vi "SubVI_HighPassFilter.vi"(7 "Interpolant Size":dbl, 8 "error in (no error)":errorcluster, 9 "high cutoff freq":dbl, 10 "EEG Desired Frequency":dbl, 11 "Channel in":T1) -> (0 "error out":errorcluster, 3 "Channel out":T1)   [LabVIEW 2020]
uses:
  <extravilib>/ChannelInstances/Stream-a[.](dbl)/)Channel.ctl
  <vilib>/Analysis/3filter.llb/Filter Passband Type.ctl
  <extravilib>/ChannelInstances/Stream-a[.](dbl)/EndpointRead.vi
  <extravilib>/ChannelInstances/Stream-a[.](dbl)/Endpoint.vi
  Global 1.vi
  <extravilib>/ChannelInstances/Stream-a[.](dbl)/)Channel.vi
  <resource>/ChannelSupport/_ChannelSupport/WaitIfNeeded.vi
  <vilib>/Analysis/NI_AALBase.lvlib
  <vilib>/ptbypt/NI_PtbyPt.lvlib
  <extravilib>/ChannelInstances/Stream-a[.](dbl).lvlib
panel:
  out "Waveform Chart 2":dbl(graph)
  out "Waveform Chart":dbl(graph)
  in  "index 2":i32
  in  "index":i32
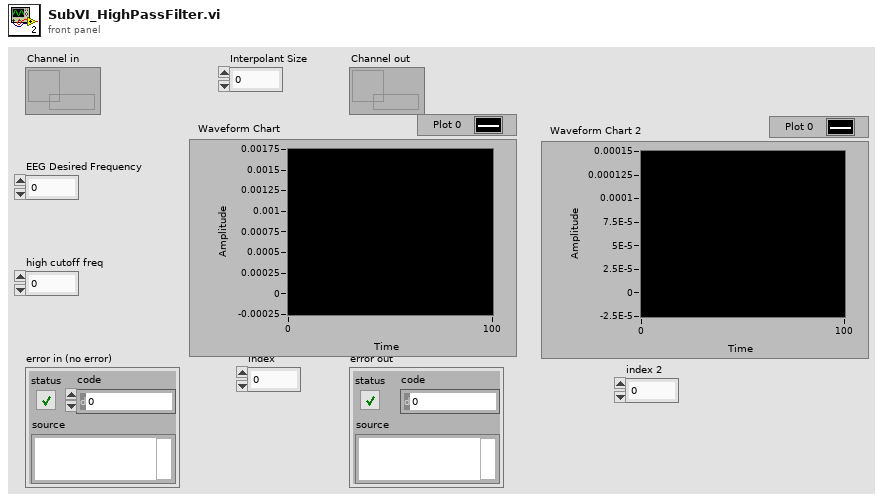
[diagram p1: front panel]
types:
  T1 = typedef "Stream-a[.](dbl).lvlib/)Channel.ctl" = refnum<queue>
  T2 = typedef "NI_AALBase.lvlib/Filter Passband Type.ctl" = enum32{"Lowpass", "Highpass", "Bandpass", "Bandstop"}
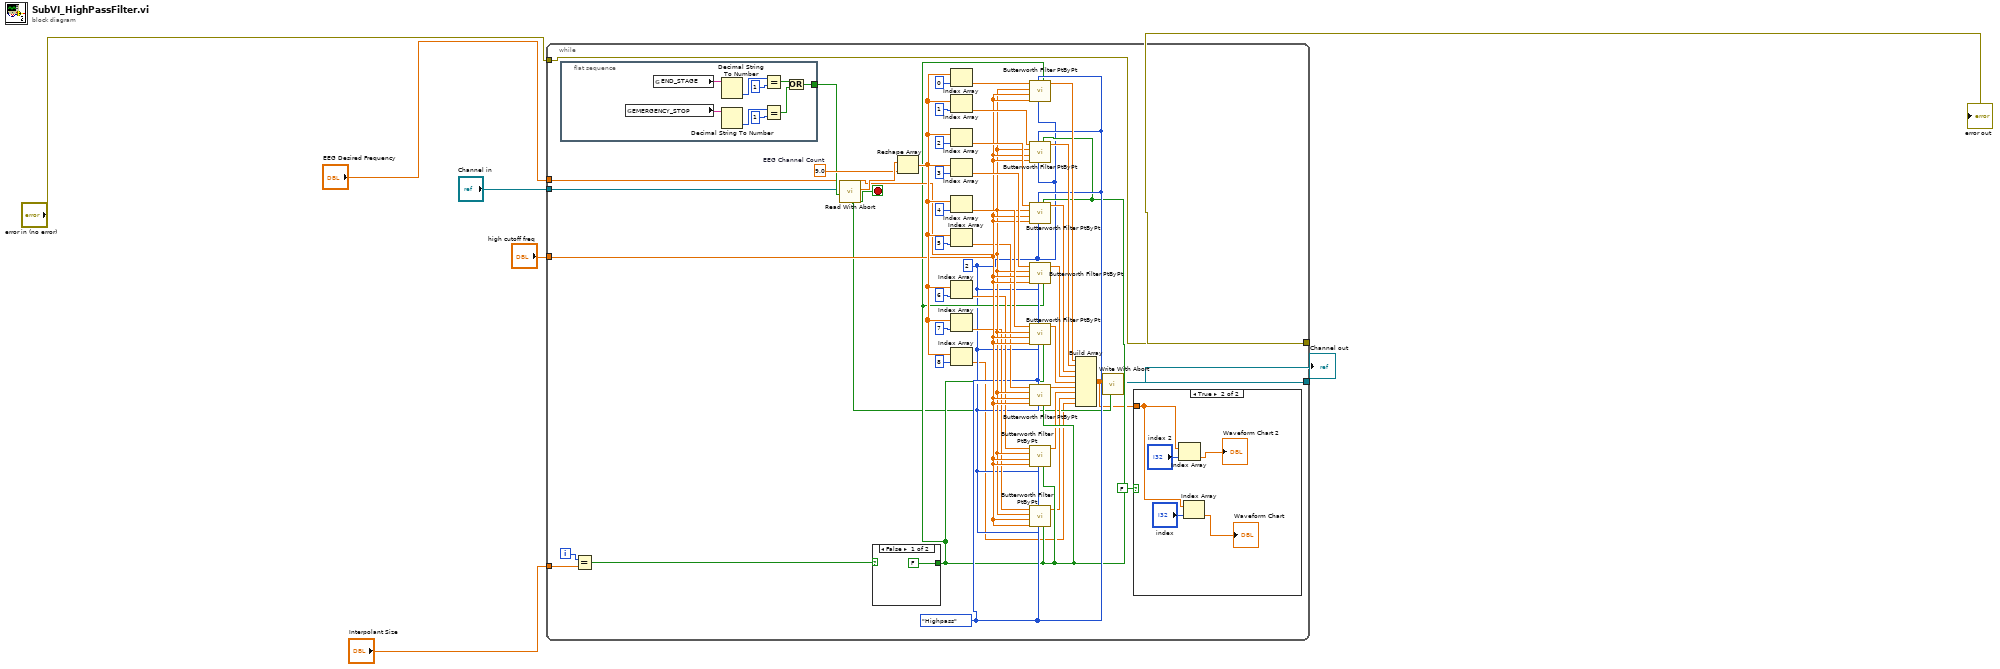
[diagram p0: block diagram]
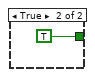
[diagram p3: hidden frame]
diagram:
  n1 = while {
    tunnel: "Channel in" -> [w29]
    tunnel: "Interpolant Size" -> [w37]
    tunnel: "EEG Desired Frequency" -> [w22]
    tunnel: "error in (no error)" -> [w30]
    tunnel: [w30] -> w7
    tunnel: "high cutoff freq" -> [w23]
    tunnel: [w11] -> w5
    i -> [w38]
    stop <- w12 stop-if-true
    w32 = 9.0  # EEG Channel Count
    w16 = 2 ("order")
    w18 = Filter_Passband_Type."Highpass" ("filter type")
    n2 = flat-sequence {
      tunnel: [w57] -> w31
      frame #0 {
        n3 = global read "Global 1.vi" "EMERGENCY_STOP"() -> (w60:string)
        n4 = global read "Global 1.vi" "END_STAGE"() -> (w65:string)
        n5 = Decimal String To Number(string=w65) -> (number=w64:i32)  [unwired: 2 in, 1 out]
        n6 = Decimal String To Number(string=w60) -> (number=w62:i32)  [unwired: 2 in, 1 out]
        n7 = Equal?(x=w64, y=1) -> (x = y?=w58:bool)
        n8 = Equal?(x=w62, y=1) -> (x = y?=w59:bool)
        n9 = Or(x=w58, y=w59) -> (x .or. y?=w57:bool)
      }
    }
    n10 = Equal?(x=w38, y=w37) -> (x = y?=w36:bool)
    n11 = call <extravilib>:"Read With Abort.vi"("abort"=w31, "channel"=w29) -> ("element"=w39:dbl[], "aborted?"=w12:bool)  [unwired: 4 in, 4 out]
    n12 = case shown="False" w36 {
      tunnel: [FALSE ("init/cont (init:F)") TRUE ("init/cont (init:F)")] -> w17
      frame False {
      }
      frame True {
      }
    }
    n13 = Reshape Array(w39, w32) -> (w24:dbl[])
    n14 = Index Array(array=w24, index=0 ("disabled index (col)")) -> (element=w48:dbl)
    n15 = Index Array(array=w24, index=1 ("disabled index (col)")) -> (element=w49:dbl)
    n16 = Index Array(array=w24, index=2 ("disabled index (col)")) -> (element=w50:dbl)
    n17 = Index Array(array=w24, index=3 ("disabled index (col)")) -> (element=w51:dbl)
    n18 = Index Array(array=w24, index=4 ("disabled index (col)")) -> (element=w35:dbl)
    n19 = Index Array(array=w24, index=5 ("disabled index (col)")) -> (element=w21:dbl)
    n20 = Index Array(array=w24, index=6 ("disabled index (col)")) -> (element=w20:dbl)
    n21 = Index Array(array=w24, index=7 ("disabled index (col)")) -> (element=w19:dbl)
    n22 = Index Array(array=w24, index=8 ("disabled index (col)")) -> (element=w10:dbl)
    n23 = call <vilib>:"Butterworth Filter PtByPt.vi"("initialize"=w17, "order"=w16, "filter type"=w18, "low cutoff freq: fl"=w23, "high cutoff freq: fh"=w23, "sampling freq: fs"=w22, "x"=w48) -> ("Filtered x"=w44:dbl)  [unwired: 2 in, 1 out]
    n24 = call <vilib>:"Butterworth Filter PtByPt.vi"("initialize"=w17, "order"=w16, "filter type"=w18, "low cutoff freq: fl"=w23, "high cutoff freq: fh"=w23, "sampling freq: fs"=w22, "x"=w49) -> ("Filtered x"=w45:dbl)  [unwired: 2 in, 1 out]
    n25 = call <vilib>:"Butterworth Filter PtByPt.vi"("initialize"=w17, "order"=w16, "filter type"=w18, "low cutoff freq: fl"=w23, "high cutoff freq: fh"=w23, "sampling freq: fs"=w22, "x"=w50) -> ("Filtered x"=w46:dbl)  [unwired: 2 in, 1 out]
    n26 = call <vilib>:"Butterworth Filter PtByPt.vi"("initialize"=w17, "order"=w16, "filter type"=w18, "low cutoff freq: fl"=w23, "high cutoff freq: fh"=w23, "sampling freq: fs"=w22, "x"=w51) -> ("Filtered x"=w47:dbl)  [unwired: 2 in, 1 out]
    n27 = call <vilib>:"Butterworth Filter PtByPt.vi"("initialize"=w17, "order"=w16, "filter type"=w18, "low cutoff freq: fl"=w23, "high cutoff freq: fh"=w23, "sampling freq: fs"=w22, "x"=w35) -> ("Filtered x"=w33:dbl)  [unwired: 2 in, 1 out]
    n28 = call <vilib>:"Butterworth Filter PtByPt.vi"("initialize"=w17, "order"=w16, "filter type"=w18, "low cutoff freq: fl"=w23, "high cutoff freq: fh"=w23, "sampling freq: fs"=w22, "x"=w21) -> ("Filtered x"=w15:dbl)  [unwired: 2 in, 1 out]
    n29 = call <vilib>:"Butterworth Filter PtByPt.vi"("initialize"=w17, "order"=w16, "filter type"=w18, "low cutoff freq: fl"=w23, "high cutoff freq: fh"=w23, "sampling freq: fs"=w22, "x"=w20) -> ("Filtered x"=w14:dbl)  [unwired: 2 in, 1 out]
    n30 = call <vilib>:"Butterworth Filter PtByPt.vi"("initialize"=w17, "order"=w16, "filter type"=w18, "low cutoff freq: fl"=w23, "high cutoff freq: fh"=w23, "sampling freq: fs"=w22, "x"=w19) -> ("Filtered x"=w13:dbl)  [unwired: 2 in, 1 out]
    n31 = Build Array(w44, w45, w46, w47, w33, w15, w14, w13, w10) -> (w9:dbl[])
    n32 = call <extravilib>:"Write With Abort.vi"("abort"=w12, "element"=w9) -> ("channel"=w11:T1)  [unwired: 6 in, 3 out]
    n33 = case shown="True" FALSE {
      tunnel: w9 -> [_ w54]
      frame False {
      }
      frame True {
        n34 = Index Array(array=w54, index="index 2") -> (element=→"Waveform Chart 2":dbl)
        n35 = Index Array(array=w54, index="index") -> (element=→"Waveform Chart":dbl)
      }
    }
  }
  "error out" <- w7
  "Channel out" <- w5
